vi "Open File+.vi"(4 "advisory dialog? (display:T)":bool=TRUE, 5 "[pattern]":string caption="[Muster]", 6 "default name":string caption="Standardname", 7 "prompt":string caption="Eingabeaufforderung", 8 "error in (not an error)":errorcluster caption="Fehler (Eingang, kein Fehler)", 9 "open mode (read-only:1)":T1(ring)=enum."read-only" caption="Öffnen-Modus (schreibgeschützt:1)", 10 "start path (Not A Path)":path=path "" caption="Startpfad (kein Pfad)", 11 "file path (\" \")":path caption="Dateipfad (\" \")") -> (0 "error out":errorcluster caption="Fehler (Ausgang)", 1 "file size (bytes)":i32 caption="Dateigröße (Byte)", 2 "file path":path caption="Dateipfad", 3 "refnum":refnum<file> caption="RefNum")   [LabVIEW 2009]
doc: "Öffnet eine existierende Datei programmgesteuert oder interaktiv unter Verwendung eines Dialogfeldes. Sie können optional eine Eingabe-Aufforderung, Standarddateinamen, Startpfad oder Filter-Muster angeben. Fehler 7 tritt auf, wenn die Datei nicht existiert. Benutzen Sie das VI zusammen mit den Mittleren \"In Datei Schreiben+\" oder \"Aus Datei Lesen+\" VIs.\n\nDateipfad ist der Pfadname der Datei. Dateipfad ist der Pfadname der Datei. Fehlercode 43 tritt auf, wenn der Anwender den Dateidialog abbricht. \n\nBeratender Dialog? Auf TRUE (Voreinstellung) setzen, wenn sie einen Dialog möchten, falls keine Datei existiert.\n\nEingabe: ist eine Meldung, die unter dem Dateidialogfenser erscheint.\n\nStandardname ist der voreingestellte Dateiname der als Standard in der Dialogbox auftaucht.\n\nStartpfad ist der Pfad, der im Dialogfenster geöffnet wird. Die Voreinstellungen ist 'Kein Pfad', was einen Zeiger auf das zuletzt geöffnete Verzeichnis bedeutet.\n\n'Öffnen-Modus' bestimmt wie die Datei geöffnet wird unter Verwendung des Refnum (Ausgang) des VIs:\n 0: Lese- und Schreibzugriff auf die Datei ist möglich.\n 1: Nur Lesezugriff möglich. Dies ist die Standardeinstellung.\n 2: Nur Schreibzugriff möglich. Entfernt keine Daten aus der Datei. (Auf nicht Mac Platformen, verhält sich diese Einstellung wie Modus 0).\n 3: Nur Schreibzugriff möglich. Entfernt keine Daten aus der Datei.\n\nMuster ist ein Vergleichsmuster, so dass nur dem Muster entsprechende Dateien angezeigt werden. Beachten Sie die Beschreibung der Dateidialog Funktionen für ausführlichere Beschreibungen.\n\nFehlereingang ist ein Cluster mit 3 Elementen (Fehler?, Code, und Quelle), das den bisherigen Fehlerstatus beschreibt, wenn bei vorher ausgeführten VIs ein Fehler aufgetreten ist. Trat kein Fehler auf, wird das VI normal ausgefürt; Trat ein Fehler auf, wird die Fehlermeldung weitergegeben. Fehler? ist TRUE wenn ein Fehler aufgetreten ist; die Voreinstellung ist FALSE. Code ist der Fehlercode; die Voreinstellung ist 0. Quelle ist in den meisten Fällen der Name des VIs oder der Funktion in der der Fehler aufgetreten ist; die Voreinstellung ist ein leerer String.\n\nNeuer Dateipfad ist der Pfad der Datei die geöffnet wird. Sie können diesen Ausgang benutzen, um den Pfad einer Datei, die Sie per Dialog öffnen, zu untersuchen. Neuer Dateipfad gibt Not A Path zurück, wenn der Benutzer im Dateidialog Abbrechen wählt.\n\nrefnum ist die Referenz zur geöffneten Datei. Der Wert ist Not A Refnum wenn die Datei nicht geöffnet werden kann.\n\nDateigröße ist die Größe der Datei in Byte und die Position des Dateiendes.\n\nFehlerausgang ist ein Cluster mit 3 Elementen (Fehler?, Code, und Quelle), das bei der Ausführung des VIs aufgetretene Fehler beschreibt. Wenn kein Eingangsfehler auftrat, wird das VI normal ausgeführt und der Fehlerausgang enthält den Fehlerstatus dieses VIs; wenn ein Eingangsfehler auftrat wird diesen an den Fehlerausgang weitergegeben."
panel:
  in  "\"%s\" not found.":string="\"%s\" nicht gefunden." caption="\"%s\" nicht gefunden."
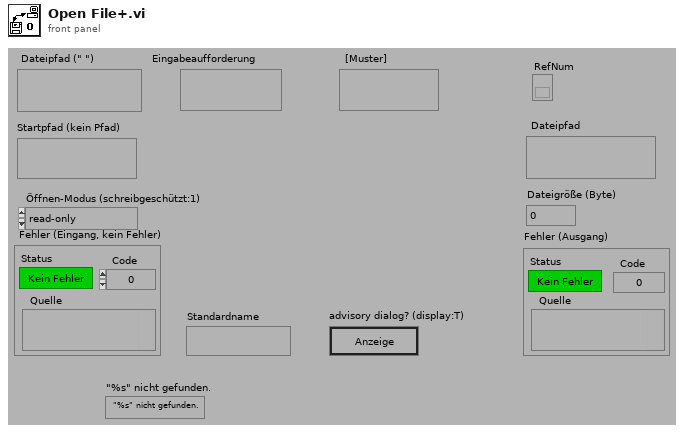
[diagram p1: front panel]
types:
  T1 = enum16{"read/write", "read-only", "write-only", "write-only (truncate)"}
  T2 = enum16{"existing file", "new file", "new or existing file", "existing dir", "new dir", "new or existing dir"}
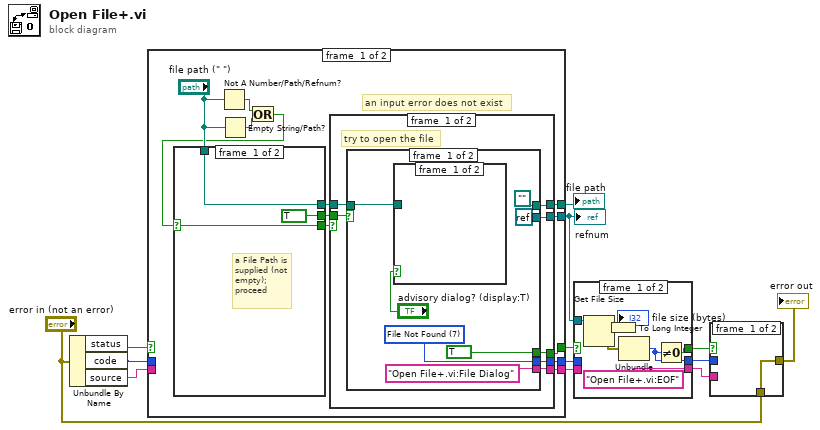
[diagram p0: block diagram]
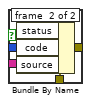
[diagram p2: hidden frame]
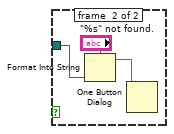
[diagram p4: hidden frame]
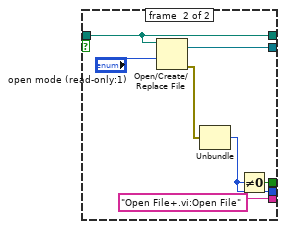
[diagram p5: hidden frame]
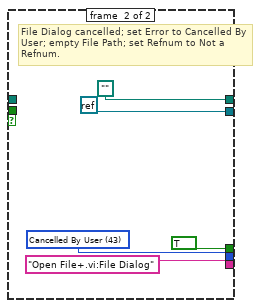
[diagram p6: hidden frame]
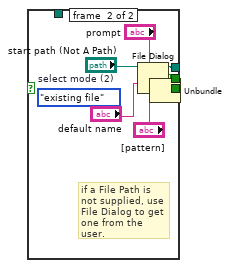
[diagram p7: hidden frame]
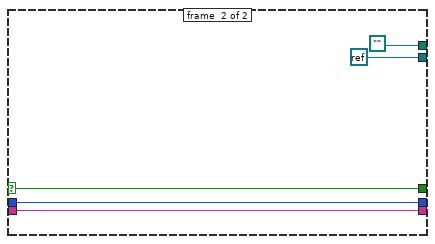
[diagram p8: hidden frame]
diagram:
  n1 = Unbundle By Name("error in (not an error)") -> ("status"=w8:bool, "code"=w5:i32, "source"=w9:string)
  n2 = case shown="False" w8 {
    selector: w8 -> [_ w68]
    tunnel: [w23 path ""] -> w13
    tunnel: [w22 refnum<k0> refnum] -> w7
    tunnel: [w21 w66] -> w12
    tunnel: [w20 w68] -> w11
    tunnel: [w19 w67] -> w10
    tunnel: w5 -> [_ w67]
    tunnel: w9 -> [_ w66]
    frame #0 {
      # "an input error does not exist"
      n3 = Not A Number/Path/Refnum?(number/path/refnum="file path (\" \")") -> (NaN/Path/Refnum?=w16:bool)
      n4 = Empty String/Path?(string/path="file path (\" \")") -> (empty?=w15:bool)
      n5 = Or(x=w16, y=w15) -> (x .or. y?=w14:bool)
      n6 = case shown="False" w14 {
        selector: w14 -> [w56 _]
        tunnel: [w56 w62] -> w25
        tunnel: [w57 w61] -> w24
        tunnel: "file path (\" \")" -> [w57 _]
        tunnel: [TRUE w59] -> w18
        frame #0 {
          # "a File Path is supplied (not empty); proceed"
        }
        frame #1 {
          (unwired) T2."existing file"  # select mode (2)
          # "if a File Path is not supplied, use File Dialog to get one from the user."
          n7 = File Dialog(6:"[pattern]", 7:"prompt", 9:"default name", 11:"start path (Not A Path)") -> (0:w58:errorcluster, 1:w62:bool, 2:w59:bool, 3:w61:path)  [unwired: 3 in]
          n8 = Unbundle(w58) -> ()  [unwired: 3 out]
        }
      }
      n9 = case shown="False" w25 {
        tunnel: w24 -> [w29 _]
        tunnel: [w28 path ""] -> w23
        tunnel: [w27 refnum<k0> refnum] -> w22
        tunnel: [w32 "Open File+.vi:File Dialog"] -> w21
        tunnel: [w31 TRUE] -> w20
        tunnel: [w26 w53] -> w19
        tunnel: w18 -> [w30 _]
        frame #0 {
          # "try to open the file"
          n10 = case shown="False" w30 {
            tunnel: ["Open File+.vi:File Dialog" "Open File+.vi:Open File"] -> w32
            tunnel: [TRUE w45] -> w31
            tunnel: w29 -> [w34 w49]
            tunnel: [path "" w49] -> w28
            tunnel: [refnum<k0> refnum w48] -> w27
            tunnel: [w35 w44] -> w26
            frame #0 {
              w35 = u16 7 items=["No Error", "Manager Argument Error", "Memory Full", "Out of Zone", "End of File", "File Already Open", "Generic File IO Error", "File Not Found", "File Permission Error", "Disk Full", "Duplicate Path", "Too Many Files Open", "Not Enabled", "Resource File Not Found", "Cannot Add Resource", "Resource Not Found", "Image Not Found", "Image Memory Error", "Pen Does Not Exist", "Config Bad Type", "Config Token Not Found", "Config Parse Error", "Config Memory Error", "Bad External Code Format", "Bad External Code Offset", "External Code Not Present", "Null Window", "Destroy Window Mixup", "Null Menu", "Print Aborted", "Bad Print Record", "Print Driver Error", "Windows Error During Print", "Memory Error During Print", "Print Dialog Error", "Generic Print Error", "Invalid Device Refnum", "Device Not Found", "Device Parameter Error", "Device Unit Error", "Can't Open Device", "Device Call Aborted", "Generic Error", "Cancelled By User"]
              n11 = case shown="True" "advisory dialog? (display:T)" {
                tunnel: w34 -> [_ w41]
                frame #0 {
                }
                frame #1 {
                  n12 = Format Into String(format string="\"%s\" not found.", w41) -> (resulting string=w42:string)  [unwired: 2 in, 1 out]
                  n13 = One Button Dialog(message=w42) -> ()  [unwired: 1 in, 1 out]
                }
              }
            }
            frame #1 {
              n14 = Open/Create/Replace File(file path (use dialog)=w49, access (0:read/write)="open mode (read-only:1)") -> (refnum out=w48:refnum<file>, error out=w46:errorcluster)  [unwired: 4 in, 1 out]
              n15 = Unbundle(w46) -> ("code"=w44:i32)  [unwired: 2 out]
              n16 = Not Equal To 0?(x=w44) -> (x != 0?=w45:bool)
            }
          }
        }
        frame #1 {
          w53 = u16 43 items=["No Error", "Manager Argument Error", "Memory Full", "Out of Zone", "End of File", "File Already Open", "Generic File IO Error", "File Not Found", "File Permission Error", "Disk Full", "Duplicate Path", "Too Many Files Open", "Not Enabled", "Resource File Not Found", "Cannot Add Resource", "Resource Not Found", "Image Not Found", "Image Memory Error", "Pen Does Not Exist", "Config Bad Type", "Config Token Not Found", "Config Parse Error", "Config Memory Error", "Bad External Code Format", "Bad External Code Offset", "External Code Not Present", "Null Window", "Destroy Window Mixup", "Null Menu", "Print Aborted", "Bad Print Record", "Print Driver Error", "Windows Error During Print", "Memory Error During Print", "Print Dialog Error", "Generic Print Error", "Invalid Device Refnum", "Device Not Found", "Device Parameter Error", "Device Unit Error", "Can't Open Device", "Device Call Aborted", "Generic Error", "Cancelled By User"]
          # "File Dialog cancelled; set Error to Cancelled By User; empty File Path; set Refnum to Not a Refnum."
        }
      }
    }
    frame #1 {
    }
  }
  "file path" <- w13
  "refnum" <- w7
  n17 = case shown="True" w11 {
    selector: w11 -> [_ w80]
    tunnel: w10 -> [_ w79]
    tunnel: w12 -> [_ w78]
    tunnel: [w76 w80] -> w4
    tunnel: [w73 w79] -> w3
    tunnel: ["Open File+.vi:EOF" w78] -> w6
    tunnel: w7 -> [w75 _]
    frame #0 {
      n18 = Get File Size(file=w75) -> (size (in bytes)=w71:i64, 0:w72:errorcluster)  [unwired: 1 in, 1 out]
      n19 = To Long Integer(number=w71) -> (32bit integer=→"file size (bytes)":i32)
      n20 = Unbundle(w72) -> ("code"=w73:i32)  [unwired: 2 out]
      n21 = Not Equal To 0?(x=w73) -> (x != 0?=w76:bool)
    }
    frame #1 {
    }
  }
  n22 = case shown="True" w4 {
    selector: w4 -> [_ w85]
    tunnel: w3 -> [_ w86]
    tunnel: w6 -> [_ w84]
    tunnel: "error in (not an error)" -> [w81 w83]
    tunnel: [w81 w82] -> w2
    frame #0 {
    }
    frame #1 {
      n23 = Bundle By Name(cluster=w83, "status"=w85, "code"=w86, "source"=w84) -> (w82:errorcluster)
    }
  }
  "error out" <- w2
